vi "GEvt-Valid Subscribers.vi"(11 "CSM Global Log Event In":T1) -> (0 "Valid":bool, 3 "CSM Global Log Event Out":T1)   [LabVIEW 2017, in "Communicable State Machine.lvlib"]
uses:
  Communicable State Machine.lvlib
  GEvt-Refs.ctl
  Typedef/_CSM_GlobalLog_MSG.ctl
  Typedef/_CSM_Response Source Message.ctl
  Typedef/_CSM_GlobalLog_MSG_TYPE.ctl
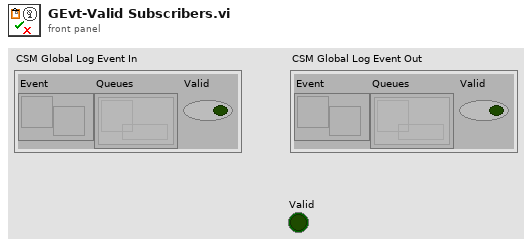
[diagram p1: front panel]
types:
  T1 = typedef "Communicable State Machine.lvlib/GEvt-Refs.ctl" = cluster{"Event":refnum<user-event>, "Queues":refnum<queue>[], "Valid":bool}
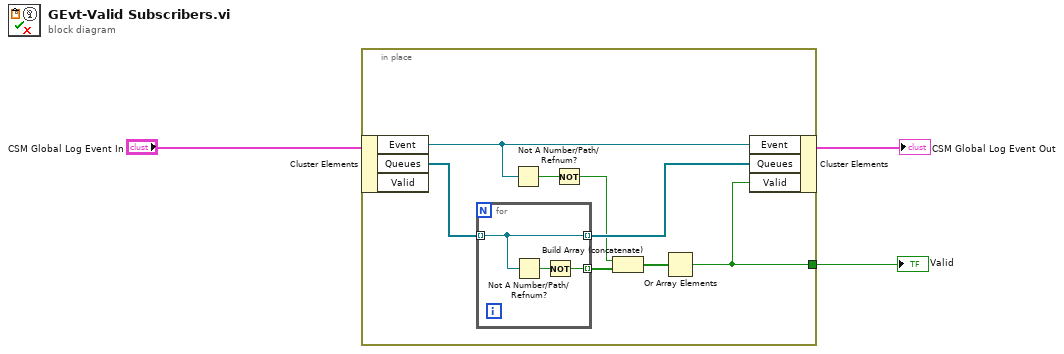
[diagram p0: block diagram]
diagram:
  n1 = in-place {
    in-place-border: [w4] -> w1
    n2 = in-place-cluster #1("CSM Global Log Event In") -> ("Event"=w9:refnum<user-event>, "Queues"=w11:refnum<queue>[])  [unwired: 1 out]
    n3 = for {
      tunnel: w11 -> [w14] mode=indexing
      tunnel: [w14] -> w10 mode=indexing
      tunnel: [w12] -> w8 mode=indexing
      n4 = Not A Number/Path/Refnum?(number/path/refnum=w14) -> (NaN/Path/Refnum?=w13:bool)
      n5 = Not(x=w13) -> (.not. x?=w12:bool)
    }
    n6 = Not A Number/Path/Refnum?(number/path/refnum=w9) -> (NaN/Path/Refnum?=w7:bool)
    n7 = Not(x=w7) -> (.not. x?=w5:bool)
    n8 = Build Array (concatenate)(w5, w8) -> (w6:bool[])
    n9 = Or Array Elements(Boolean array=w6) -> (logical OR=w4:bool)
    n10 = in-place-cluster #1("Event"=w9, "Queues"=w10, "Valid"=w4) -> (→"CSM Global Log Event Out":T1)
  }
  "Valid" <- w1
